vi "Destroy.vi"(0 "reference in":refnum<class "subject.lvclass">, 5 "error in (no error)":errorcluster) -> (14 "reference out":refnum<class "subject.lvclass">, 19 "error out":errorcluster)   [LabVIEW 2015, in "subject.lvclass"]
doc: "Destructor."
uses:
  subject.lvclass
  <vilib>/addons/_AddQ/G#Object/G#Object.lvclass
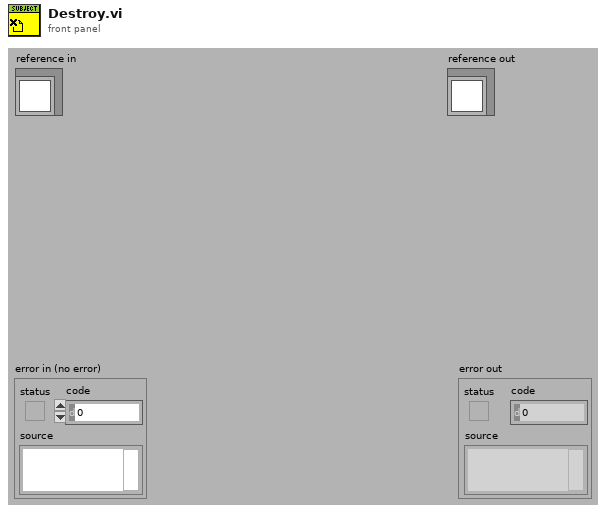
[diagram p1: front panel]
types:
  T1 = typedef "subject.lvclass/ObjectAttributes.ctl" = cluster{"MyAttribute":dbl, "data":cluster{"Ve_warm":dbl[], "time_warm":dbl[], "name":string, "phase":dbl[], "VCO2":dbl[], "VO2":dbl[], "PetCO2":dbl[], "RQ":dbl[], "HR":dbl[], "Ve_warm_inter":dbl[], "time_warm_inter":dbl[], "Ve_exer":dbl[], "time_exer":dbl[], "Ve_exer_inter":dbl[], "time_exer_inter":dbl[], "Ve":dbl[], "time":dbl[]}, "results_5l":cluster{"EOV":bool, "osci_amplitude":dbl[], "osci_width":dbl[], "peak_location":dbl[], "threshold":dbl, "width":i32}, "results_15percent":cluster{"EOV":bool, "osci_amplitude":dbl[], "osci_width":dbl[], "peak_location":dbl[], "threshold":dbl, "width":i32}, "supportData":cluster{"peaksAmplitude":dbl[], "iPeaksLocation":dbl[], "valesAmplitude":dbl[], "iValesLocation":dbl[], "threshold":dbl, "meanAmpl_warm":i32, "#_peaks":i32, "width":i32}, "results_user_selection":cluster{"EOV":bool, "osci_amplitude":dbl[], "osci_width":dbl[], "peak_location":dbl[], "threshold":dbl, "width":i32}}
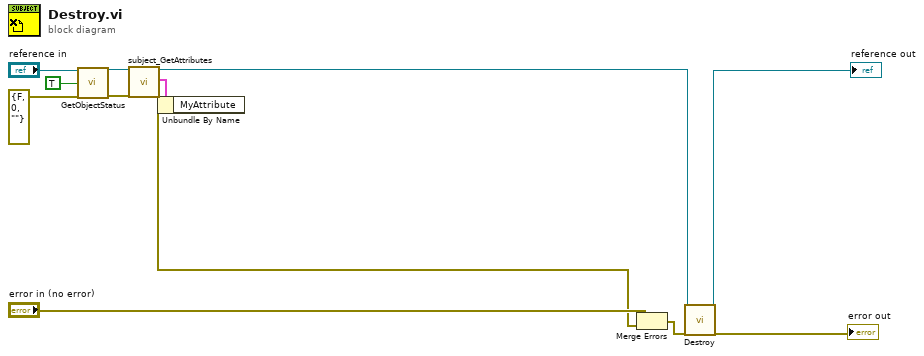
[diagram p0: block diagram]
diagram:
  n1 = call-dynamic "GetObjectStatus.vi"("reference in"="reference in", "simple info (F)"=TRUE ("simple info"), "error in (no error)"=errorcluster {"status"=FALSE, "code"=0, "source"=""}) -> ("reference out"=w5:refnum<class "subject.lvclass">, "error out"=w6:errorcluster)  [unwired: 5 in, 10 out]
  n2 = call "subject_GetAttributes.vi"("reference in"=w5, "error in (no error)"=w6) -> ("reference out"=w4:refnum<class "subject.lvclass">, "attributes"=w3:T1, "error out"=w7:errorcluster)  [unwired: 14 in, 1 out]
  n3 = Unbundle By Name(w3) -> ()  [unwired: 1 out]
  n4 = Merge Errors("error in (no error)", w7) -> (w11:errorcluster)
  n5 = call-parent "Destroy.vi"("reference in"=w4, "error in (no error)"=w11) -> ("reference out"=→"reference out":refnum<class "subject.lvclass">, "error out"=→"error out":errorcluster)  [unwired: 16 in]
